vi "DamnYankeeFPGA_analog_test.vi"() -> ()   [LabVIEW 2013]
uses:
  <vilib>/eio/EIONode/EIONode.xnode
  <vilib>/rvi/DataTransferAndStorage/Container/XNode/niFpgaContainer.xnode
  <vilib>/rvi/eio/common/nirviEmuTemplateMethod_errors.vi
panel:
  in  "Count(uSec)":u32
  out "largest value":u16
  out "Waveform Chart":u16(graph)
  out "ConnectorA/AI2":u16
  out "Loop counter":i32
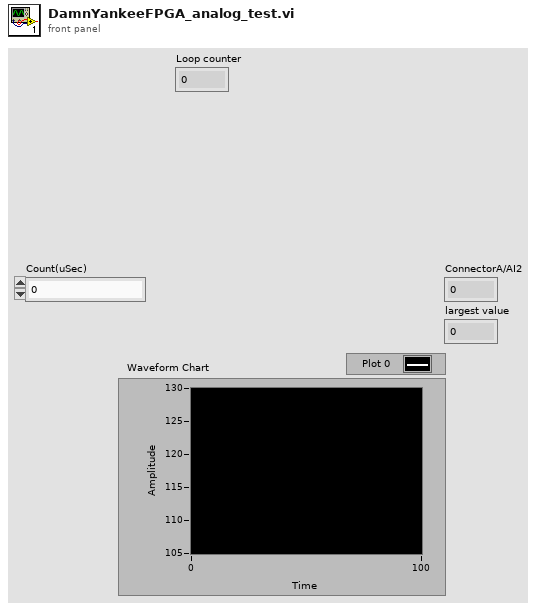
[diagram p1: front panel]
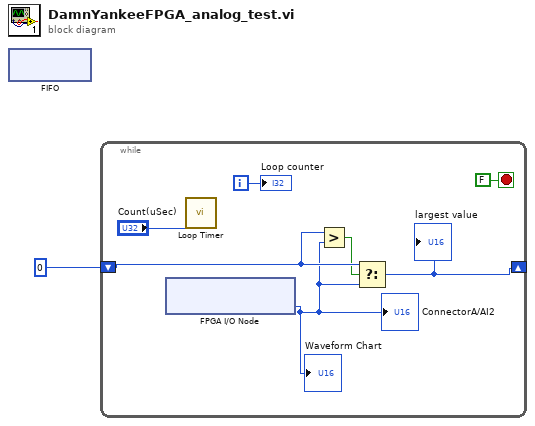
[diagram p0: block diagram]
diagram:
  n1 = xnode "FIFO"() -> ()  [unwired: 1 in, 1 out]
  n2 = while {
    shift-right: [w6] -> _
    shift-left: u16 0 ("ConnectorA/AI2") -> [w5]
    i -> [w7]
    stop <- FALSE stop-if-true
    n3 = xnode "FPGA I/O Node"() -> ("ConnectorA/AI2"=w4:u16)  [unwired: 1 in, 1 out]
    "ConnectorA/AI2" <- w4
    "Waveform Chart" <- w4
    n4 = call "Loop Timer"("Count(uSec)"="Count(uSec)") -> ()  [unwired: 1 out]
    n5 = Greater?(x=w5, y=w4) -> (0:w3:bool)
    n6 = Select(t=w5, s=w3, f=w4) -> (s? t:f=w6:u16)
    "largest value" <- w6
    "Loop counter" <- w7
  }
